vi "Close Hardware.vi"(8 "error in (no error)":errorcluster, 11 "Inst.Magneto in":refnum<class "Inst.Magneto.lvclass">) -> (0 "error out":errorcluster, 3 "Inst.Magneto out":refnum<class "Inst.Magneto.lvclass">)   [LabVIEW 2019, in "Inst.Magneto.lvclass"]
uses:
  Inst.Magneto.lvclass
  Inst.Magneto.lvclass/Inst.Magneto.ctl
  <userlib>/Levylab/Instrument Framework/Instrument Types/VSource/Instrument.VSource.lvclass
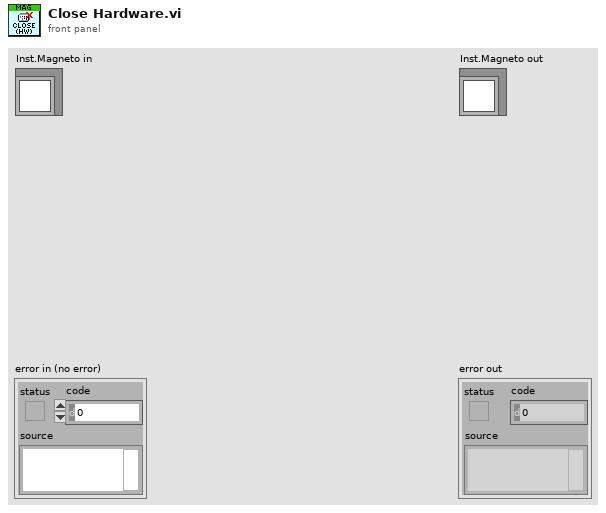
[diagram p1: front panel]
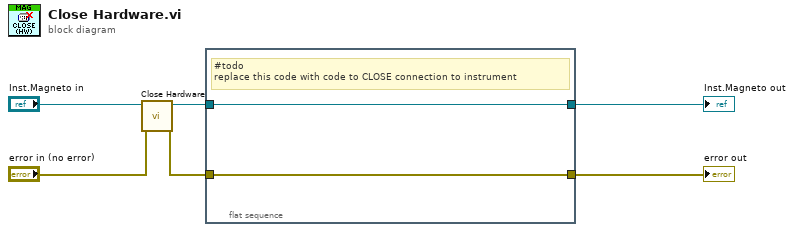
[diagram p0: block diagram]
diagram:
  n1 = call-parent "Close Hardware.vi"("error in (no error)"="error in (no error)", "Instrument in"="Inst.Magneto in") -> ("error out"=w4:errorcluster, "Instrument out"=w2:refnum<class "Inst.Magneto.lvclass">)  [unwired: 8 in]
  n2 = flat-sequence {
    tunnel: w4 -> [w8]
    tunnel: [w8] -> w3
    tunnel: w2 -> [w7]
    tunnel: [w7] -> w1
    frame #0 {
      # "#todo\nreplace this code with code to CLOSE connection to instrument"
    }
  }
  "error out" <- w3
  "Inst.Magneto out" <- w1
